vi "Initialize FPGA.vi"(8 "error in":errorcluster) -> (0 "error out":errorcluster, 3 "FPGA Out":T1)   [LabVIEW 2012]
uses:
  <vilib>/rvi/interface/nirviOpenFPGA/nirviOpenFPGA.xnode
  <vilib>/rvi/interface/nirviMethod/nirviMethod.xnode
  FPGA Bitfiles/AutonomousUnicyc_FPGATarget_9870InterfaceDMA_YGYsAJvlDFc.lvbitx
  Program Files (x86)/National Instruments/LabVIEW 2012/examples/CompactRIO/Module Specific/NI 987x/Serial Loopback/VIs/9870 Interface DMA (FPGA).vi
  <vilib>/FPGAPlugInAG/cRIO-9113/niLvFpga_Open_cRIO-9113.vi
  <vilib>/FPGAPlugInAG/cRIO-9113/niLvFpga_Reset_cRIO-9113.vi
  <vilib>/rvi/interface/nirviMethod/StockFPGA_InlinedMethodWaitForSingleIRQ.vi
  <vilib>/FPGAPlugInAG/cRIO-9113/niLvFpga_WaitOnIrq_cRIO-9113.vi
  <vilib>/FPGAPlugInAG/cRIO-9113/niLvFpga_Run_cRIO-9113.vi
  FPGA Example Files/901x DMA FPGA Reference.ctl
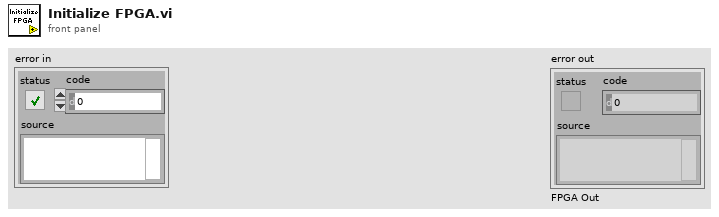
[diagram p1: front panel]
types:
  T1 = typedef "901x DMA FPGA Reference.ctl" = refnum<k20>
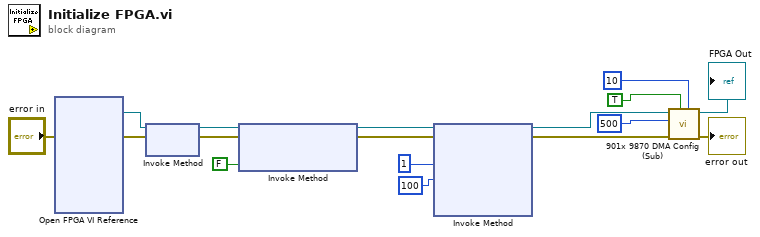
[diagram p0: block diagram]
diagram:
  n1 = xnode "Open FPGA VI Reference"("error in"="error in") -> ("FPGA VI Reference Out"=w17:refnum<k20>, "error out"=w16:errorcluster)  [unwired: 1 in]
  n2 = xnode "Invoke Method"("FPGA VI Reference In"=w17, "error in"=w16) -> ("FPGA VI Reference Out"=w13:refnum<k20>, "error out"=w14:errorcluster)
  n3 = xnode "Invoke Method"("FPGA VI Reference In"=w13, "error in"=w14, "Wait Until Done (F)"=FALSE) -> ("FPGA VI Reference Out"=w10:refnum<k20>, "error out"=w11:errorcluster)
  n4 = xnode "Invoke Method"("FPGA VI Reference In"=w10, "error in"=w11, "IRQ Number(s)"=1, "Timeout (ms)"=100) -> ("FPGA VI Reference Out"=w1:refnum<k20>, "error out"=w6:errorcluster)  [unwired: 2 out]
  n5 = call "901x 9870 DMA Config (Sub).vi"("EOS Byte"=10, "Enable EOS"=TRUE, "error in"=w6, "Byte Timeout"=500, "FPGA In"=w1) -> ("error out"=→"error out":errorcluster, "FPGA Out"=→"FPGA Out":T1)  [unwired: 5 in]
